vi "DriveExecute.vi"(8 "error in (no error)":errorcluster) -> (0 "error out":errorcluster)   [LabVIEW 2023]
doc: "Execute for Drie\n\nClosed control loop for drive\n\ninput: \n error in (cluster)\n\noutput:\n error out (cluster)"
uses:
  <vilib>/Rock Robotics/WPI/ThirdParty/JAS_Junk/TrajLib/LinearFilter_ResetToValue.vi
  <vilib>/Rock Robotics/WPI/ThirdParty/JAS_Junk/TrajLib/LinearFilter_Calculate.vi
  DriveGlobal.vi
  <vilib>/Rock Robotics/WPI/ThirdParty/JAS_Junk/TrajLib/LinearFilter_MovingAverage.vi
  <vilib>/Rock Robotics/WPI/ThirdParty/JAS_Junk/TrajLib/LinearFilter_LowPassBW1.vi
  <vilib>/Rock Robotics/WPI/ThirdParty/JAS_Junk/TrajLib/LinearFilter_LowPassBW2.vi
  <vilib>/Rock Robotics/WPI/ThirdParty/JAS_Junk/TrajLib/LinearFilter_HighPassBW1.vi
  <vilib>/Rock Robotics/WPI/ThirdParty/JAS_Junk/TrajLib/LinearFilter_HighPassBW2.vi
  <vilib>/Rock Robotics/WPI/ThirdParty/JAS_Junk/TrajLib/Trajectory_Library.lvlib
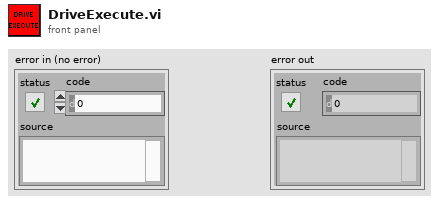
[diagram p1: front panel]
types:
  T1 = typedef "Trajectory_Library.lvlib/CHASSIS_SPEEDS.ctl" = cluster{"vX":dbl, "vY":dbl, "vOmega":dbl}
  T2 = typedef "Trajectory_Library.lvlib/SWERVE_DRIVE_KINEMATICS.ctl" = cluster{"NumModules":i32, "InverseKinematics":T3, "ForwardKinematics":T3, "Modules":T4[], "PrevCoR":T4, "SavedModuleStates":T5[]}
  T3 = typedef "NI_Matrix.lvlib/RealMatrix.ctl" = dbl[][]
  T4 = typedef "Trajectory_Library.lvlib/TRANSLATION2D.ctl" = cluster{"X":dbl, "Y":dbl}
  T5 = typedef "Trajectory_Library.lvlib/SWERVE_DRIVE_MODULE_STATE.ctl" = cluster{"Speed":dbl, "Angle":T6}
  T6 = typedef "Trajectory_Library.lvlib/ROTATION2D.ctl" = cluster{"VALUE":dbl, "COS":dbl, "SIN":dbl}
  T7 = typedef "Trajectory_Library.lvlib/SWERVE_DRIVE_MODULE_POSITION.ctl" = cluster{"Distance":dbl, "Angle":T6, "P":bool}
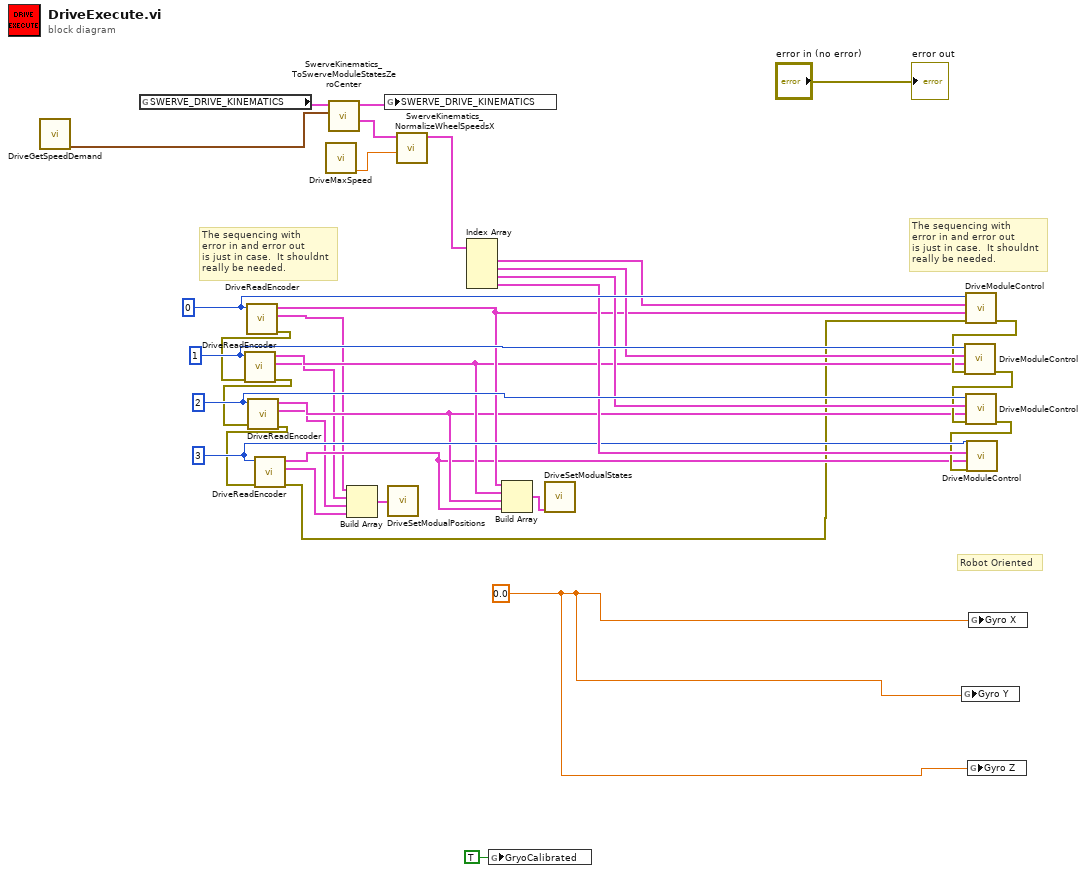
[diagram p0: block diagram]
diagram:
  w2 = 0.0
  w30 = 0 ("ModualNamePrefix")
  w29 = 1 ("ModualNamePrefix")
  w28 = 2 ("ModualNamePrefix")
  w23 = 3 ("ModualNamePrefix")
  # "Robot Oriented"
  # "The sequencing with\nerror in and error out\nis just in case.  It shouldnt\nreally be needed."
  # "The sequencing with\nerror in and error out\nis just in case.  It shouldnt\nreally be needed."
  n1 = call "DriveGetSpeedDemand.vi"() -> ("ChassisSpeedDemand"=w32:T1)  [unwired: 8 in, 3 out]
  n2 = global read "DriveGlobal.vi" "SWERVE_DRIVE_KINEMATICS"() -> (w33:T2)
  n3 = call "DriveReadEncoder.vi"("ModualNamePrefix"=w30) -> ("error out"=w9:errorcluster, "SWERVE_DRIVE_MODULE_POSITION"=w15:T7, "SWERVE_DRIVE_MODULE_STATE"=w19:T5)  [unwired: 8 in]
  n4 = call "DriveReadEncoder.vi"("error in"=w9, "ModualNamePrefix"=w29) -> ("error out"=w8:errorcluster, "SWERVE_DRIVE_MODULE_POSITION"=w14:T7, "SWERVE_DRIVE_MODULE_STATE"=w18:T5)  [unwired: 7 in]
  n5 = call "DriveReadEncoder.vi"("error in"=w8, "ModualNamePrefix"=w28) -> ("error out"=w7:errorcluster, "SWERVE_DRIVE_MODULE_POSITION"=w13:T7, "SWERVE_DRIVE_MODULE_STATE"=w17:T5)  [unwired: 7 in]
  n6 = call "DriveReadEncoder.vi"("error in"=w7, "ModualNamePrefix"=w23) -> ("error out"=w6:errorcluster, "SWERVE_DRIVE_MODULE_POSITION"=w12:T7, "SWERVE_DRIVE_MODULE_STATE"=w16:T5)  [unwired: 7 in]
  n7 = call "DriveMaxSpeed.vi"() -> ("Max Speed (m/sec)"=w4:dbl)  [unwired: 10 in, 1 out]
  n8 = call <vilib>:"SwerveKinematics_ToSwerveModuleStatesZeroCenter.vi"("ChassisSpeeds"=w32, "in SWERVE_DRIVE_KINEMATICS"=w33) -> ("ModuleStates"=w5:T5[], "out SWERVE_DRIVE_KINEMATICS"=w31:T2)  [unwired: 8 in]
  n9 = Build Array(w15, w14, w13, w12) -> (w10:T7[])
  n10 = global write "DriveGlobal.vi" "SWERVE_DRIVE_KINEMATICS"(w31) -> ()
  n11 = call "DriveSetModualPositions.vi"("Swerve_Drive_Modual_Position"=w10) -> ()  [unwired: 11 in]
  n12 = call <vilib>:"SwerveKinematics_NormalizeWheelSpeedsX.vi"("AttainableMaxSpeed"=w4, "in WheelStates"=w5) -> ("out WheelStates"=w3:T5[])  [unwired: 9 in]
  n13 = Index Array(array=w3) -> (element #1=w24:T5, element #2=w27:T5, element #3=w26:T5, element #4=w25:T5)  [unwired: 4 in]
  n14 = global write "DriveGlobal.vi" "GryoCalibrated"(TRUE ("GryoCalibrated")) -> ()
  n15 = Build Array(w19, w18, w17, w16) -> (w11:T5[])
  n16 = call "DriveSetModualStates.vi"("Swerve__Drive_Modual_States"=w11) -> ()  [unwired: 11 in]
  n17 = global write "DriveGlobal.vi" "Gyro Y"(w2) -> ()
  n18 = call "DriveModuleControl.vi"("error in"=w6, "Actual State"=w19, "Desired State"=w24, "ModualNamePrefix"=w30) -> ("error out"=w22:errorcluster)  [unwired: 7 in]
  n19 = call "DriveModuleControl.vi"("error in"=w22, "Actual State"=w18, "Desired State"=w27, "ModualNamePrefix"=w29) -> ("error out"=w21:errorcluster)  [unwired: 7 in]
  n20 = call "DriveModuleControl.vi"("error in"=w21, "Actual State"=w17, "Desired State"=w26, "ModualNamePrefix"=w28) -> ("error out"=w20:errorcluster)  [unwired: 7 in]
  n21 = call "DriveModuleControl.vi"("error in"=w20, "Actual State"=w16, "Desired State"=w25, "ModualNamePrefix"=w23) -> ()  [unwired: 7 in, 1 out]
  n22 = global write "DriveGlobal.vi" "Gyro Z"(w2) -> ()
  n23 = global write "DriveGlobal.vi" "Gyro X"(w2) -> ()
  "error out" <- "error in (no error)"
